vi "Do.vi"(8 "error in (no error)":errorcluster, 10 "Actor in":refnum<class "Actor.lvclass">, 11 "Set Sart Cameras Msg":refnum<class "Set Sart Cameras Msg.lvclass">) -> (0 "error out":errorcluster, 2 "Actor out":refnum<class "Actor.lvclass">)   [LabVIEW 2014, in "HIJ 3 Alignment Cams App.lvlib" / "Set Sart Cameras Msg.lvclass"]
doc: "This VI delivers the message to the actor by calling the appropriate method(s) on the actor."
uses:
  Set Sart Cameras Msg.lvclass
  <vilib>/ActorFramework/Actor/Actor.lvclass
  HIJ 3 Aligment Cams Launcher/HIJ 3 Aligment Cams Launcher.lvclass
  Set Sart Cameras Msg.lvclass/Set Sart Cameras Msg.ctl
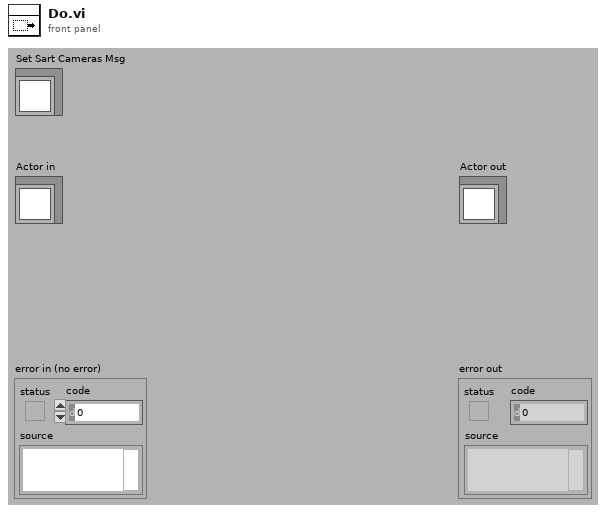
[diagram p1: front panel]
types:
  T1 = typedef "IMAQdx.ctl" = refnum<k21>
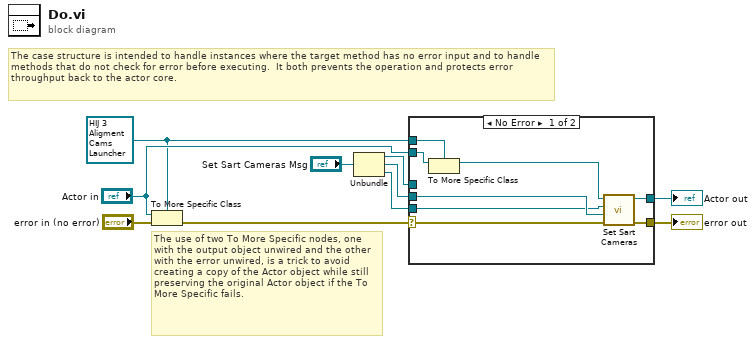
[diagram p0: block diagram]
diagram:
  w4 = refnum<class "HIJ 3 Aligment Cams Launcher.lvclass"> refnum ("Actor in")
  # "The use of two To More Specific nodes, one with the output object unwired and the other with the error unwired, is a trick to avoid creating a copy of the Actor object while still preserving the original Actor object if the To More Specific fails."
  # "The case structure is intended to handle instances where the target method has no error input and to handle methods that do not check for error before executing.  It both prevents the operation and protects error throughput back to the actor core."
  n1 = To More Specific Class(target class=w4, reference="Actor in", error in="error in (no error)") -> (error out=w8:errorcluster)  [unwired: 1 out]
  n2 = Unbundle("Set Sart Cameras Msg") -> (w3:T1, w2:T1, w1:T1)
  n3 = case shown="No Error" w8 {
    selector: w8 -> [w16 w20]
    tunnel: [w18 w20] -> w7
    tunnel: [w17 w19] -> w6
    tunnel: "Actor in" -> [w15 w19]
    tunnel: w4 -> [w14 _]
    tunnel: w3 -> [_ _]
    tunnel: w2 -> [w12 _]
    tunnel: w1 -> [w11 _]
    frame No Error {
      n4 = To More Specific Class(target class=w14, reference=w15) -> (specific class reference=w13:refnum<class "HIJ 3 Aligment Cams Launcher.lvclass">)  [unwired: 1 in, 1 out]
      n5 = call "Set Sart Cameras.vi"("error in (no error)"=w16, "Camera 3"=w12, "Camera 2"=w11, "HIJ 4 Aligment Cams Launcher in"=w13) -> ("error out"=w18:errorcluster, "HIJ 4 Aligment Cams Launcher out"=w17:refnum<class "HIJ 3 Aligment Cams Launcher.lvclass">)  [unwired: 6 in]
    }
    frame Error {
      # "If type check fails, pass the original object out again."
    }
  }
  "error out" <- w7
  "Actor out" <- w6
